vi "260520_demo_test_tryout.vi"() -> ()   [LabVIEW 2022 SP3]
uses:
  <vilib>/express/express analysis/Spectral/Block/exnSpectralBlock spectral measurements peak poly.vi
  <vilib>/express/express analysis/Spectral/Block/exnSpectralBlock spectral measurements peak DDT.vi
  <vilib>/express/express analysis/Spectral/XNode/ExpressSpectralMeasurementsBlockNode.xnode
panel:
  out "疊層訊號 2":dynamicdata(graph)
  out "SPC ALARM":bool
  out "Numeric":i32
  out "疊層訊號":dbl[][](graph)
  out "C1-3":dynamicdata(graph)
  out "C1-2":dynamicdata(graph)
  out "C1-1":dynamicdata(graph)
  out "C1-0":dynamicdata(graph)
  out "appended path":path
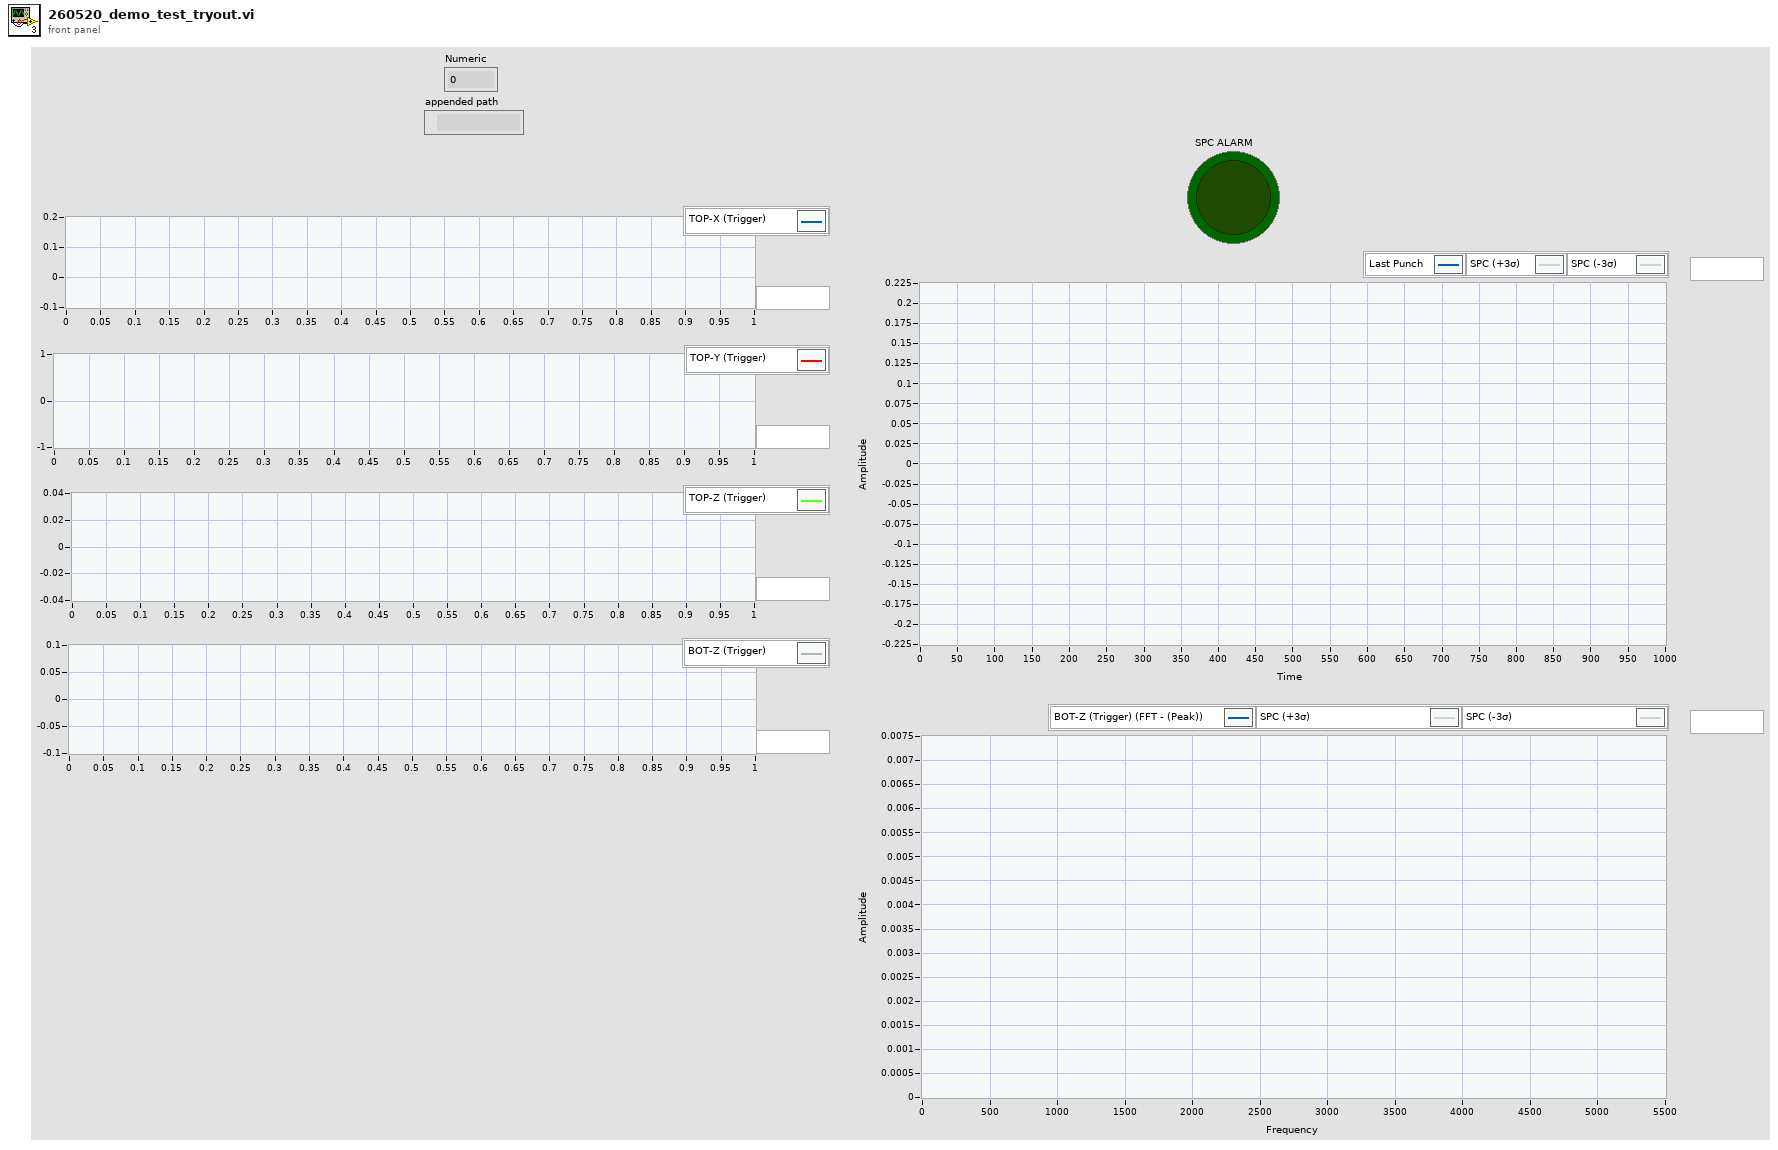
[diagram p1: front panel]
types:
  T1 = cluster{"averaging mode":u16, "weighting mode":u16, "number of averages":u32}
  T2 = cluster{"dB On (F)":bool, "unwrap phase (F)":bool, "convert to degree (F)":bool}
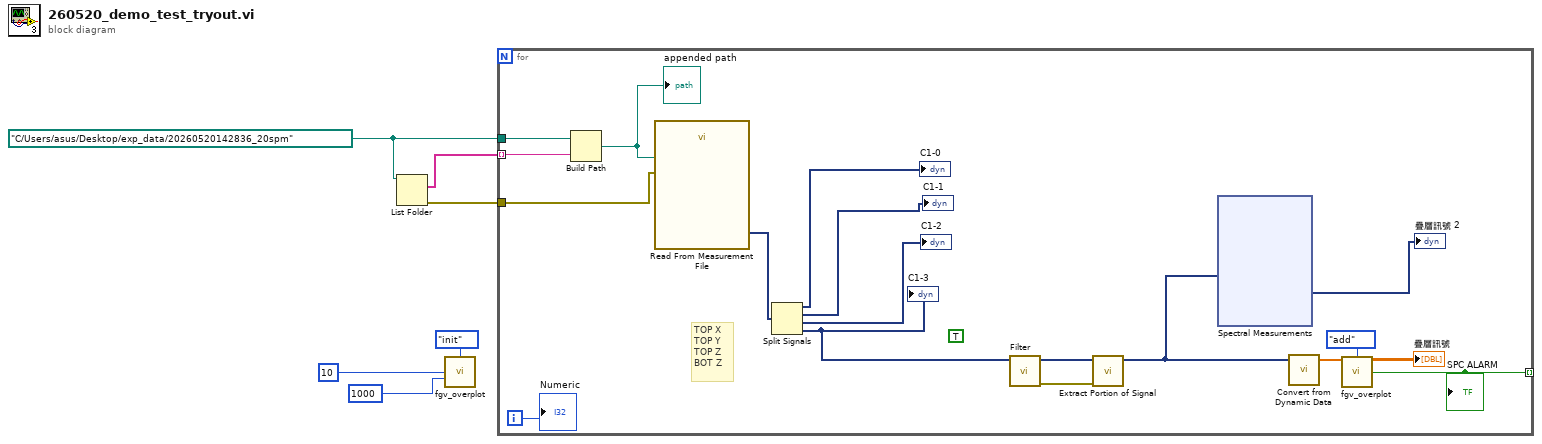
[diagram p0: block diagram]
diagram:
  w6 = path "C:/Users/asus/Desktop/exp_data/20260520142836_20spm" ("base path")
  n1 = List Folder(path=w6) -> (filenames=w4:string[], error out=w5:errorcluster)  [unwired: 3 in, 2 out]
  n2 = call "fgv_overplot.vi"("function (default: show)"=enum16{"init", "add"}."init", "num for avg"=u32 10, "total samples"=u32 1000 ("num for avg")) -> ()  [unwired: 10 in, 3 out]
  n3 = for {
    tunnel: w6 -> [w24]
    tunnel: w5 -> [w23]
    tunnel: w4 -> [w22] mode=indexing
    tunnel: [w10] -> _ mode=indexing
    i -> [w11]
    (unwired) TRUE
    # "TOP X\nTOP Y\nTOP Z\nBOT Z"
    n4 = Build Path(base path=w24, name or relative path=w22) -> (appended path=w21:path)
    "appended path" <- w21
    n5 = call "Read From Measurement File"("error in (no error)"=w23, "Filename"=w21) -> ("Signals"=w20:dynamicdata)  [unwired: 4 in, 5 out]
    n6 = Split Signals(w20) -> (→"C1-0":dynamicdata, →"C1-1":dynamicdata, →"C1-2":dynamicdata, w14:dynamicdata)  [unwired: 4 in]
    "C1-3" <- w14
    n7 = call "Filter"("Signal"=w14) -> ("error out"=w7:errorcluster, "Filtered Signal"=w13:dynamicdata)  [unwired: 9 in]
    n8 = call "Extract Portion of Signal"("error in (no error)"=w7, "Signals"=w13) -> ("Section"=w8:dynamicdata)  [unwired: 8 in, 1 out]
    n9 = xnode "Spectral Measurements"("Signals"=w8) -> ("FFT - (Peak)"=→"疊層訊號 2":dynamicdata)  [unwired: 1 in, 2 out]
    n10 = call "Convert from Dynamic Data"("Dynamic Data Type"=w8) -> ("Array"=w15:dbl[])  [unwired: 3 in]
    n11 = call "fgv_overplot.vi"("Data in"=w15, "function (default: show)"=enum16{"init", "add"}."add") -> ("Plot"=→"疊層訊號":dbl[][], "SPC ALARM"=w10:bool)  [unwired: 11 in, 1 out]
    "SPC ALARM" <- w10
    "Numeric" <- w11
  }
